vi "End.vi"(8 "error in (no error)":errorcluster, 11 "Server in":refnum<class "Server.lvclass">) -> (0 "error out":errorcluster, 3 "Server out":refnum<class "Server.lvclass">)   [LabVIEW 2018, in "Server.lvclass"]
uses:
  Server.lvclass
  Comm/Stream/Stream.lvclass
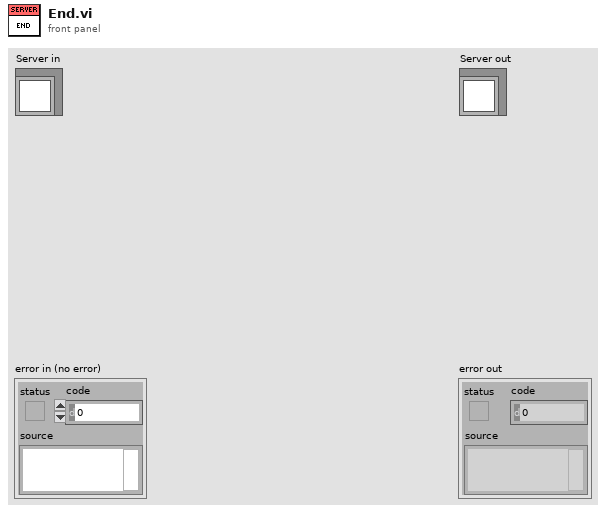
[diagram p1: front panel]
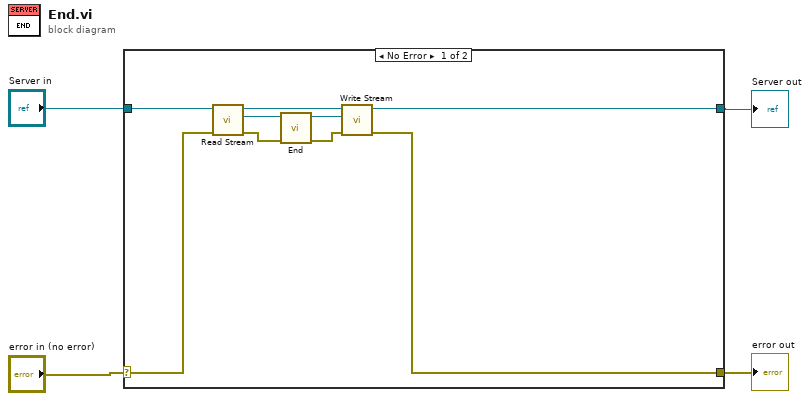
[diagram p0: block diagram]
diagram:
  n1 = case shown="No Error" "error in (no error)" {
    selector: "error in (no error)" -> [w11 w15]
    tunnel: [w5 w15] -> w1
    tunnel: [w6 w14] -> w2
    tunnel: "Server in" -> [w13 w14]
    frame No Error {
      n2 = call-dynamic "Read Stream.vi"("error in (no error)"=w11, "Server in"=w13) -> ("error out"=w10:errorcluster, "Stream.lvclass"=w12:refnum<class "Stream.lvclass">, "Server out"=w7:refnum<class "Server.lvclass">)  [unwired: 7 in]
      n3 = call-dynamic "End.vi"("error in (no error)"=w10, "Stream in"=w12) -> ("error out"=w8:errorcluster, "Stream out"=w9:refnum<class "Stream.lvclass">)  [unwired: 8 in]
      n4 = call-dynamic "Write Stream.vi"("error in (no error)"=w8, "Stream.lvclass"=w9, "Server in"=w7) -> ("error out"=w5:errorcluster, "Server out"=w6:refnum<class "Server.lvclass">)  [unwired: 7 in]
    }
    frame Error {
    }
  }
  "error out" <- w1
  "Server out" <- w2
